vi "test21-RegisterInterruptFromNonCSM.vi"(8 "error in (no error)":errorcluster, 11 "TestCase in":refnum<class "testcase-CSMBroadcast.lvclass">) -> (0 "error out":errorcluster, 3 "TestCase out":refnum<class "testcase-CSMBroadcast.lvclass">)   [LabVIEW 2017, in "testcase-CSMBroadcast.lvclass"]
uses:
  testcase-CSMBroadcast.lvclass
  <vilib>/addons/_JKI Toolkits/VI Tester/TestCase.llb/TestCase.lvclass
  src/user.lib/_NEVSTOP/Communicable State Machine(CSM)/Communicable State Machine.lvlib
  CSM/CSM-Testcase.lvlib
  C:/Program Files (x86)/National Instruments/LabVIEW 2017/vi.lib/addons/_JKI Toolkits/VI Tester/TestCase.llb/TestCase.lvclass
panel:
  out "output cluster":T1
  out "LoopCount":i32
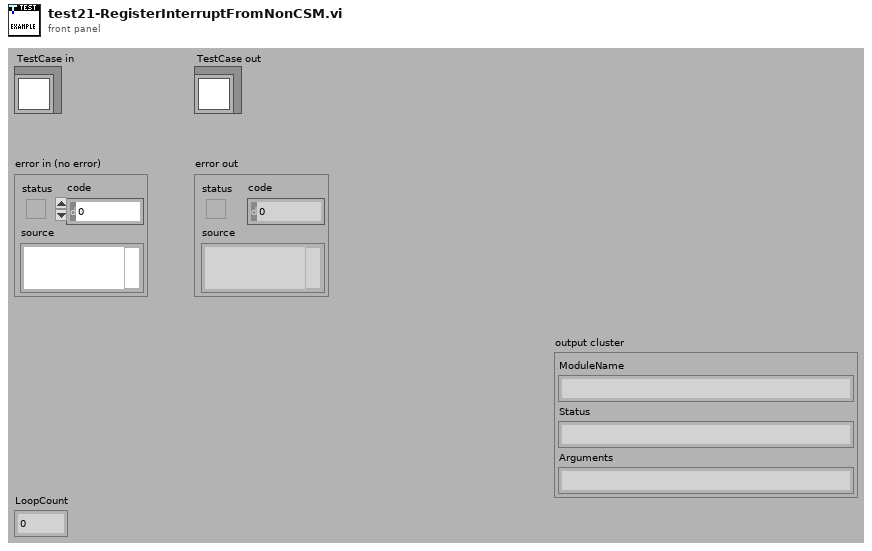
[diagram p1: front panel]
types:
  T1 = cluster{"ModuleName":string, "Status":string, "Arguments":string}
  T2 = cluster{"Status Event":refnum<user-event>, "Interrupt Event":refnum<user-event>}
  T3 = cluster{"cluster":cluster{"ModuleName":string, "Status":string, "Arguments":string}}
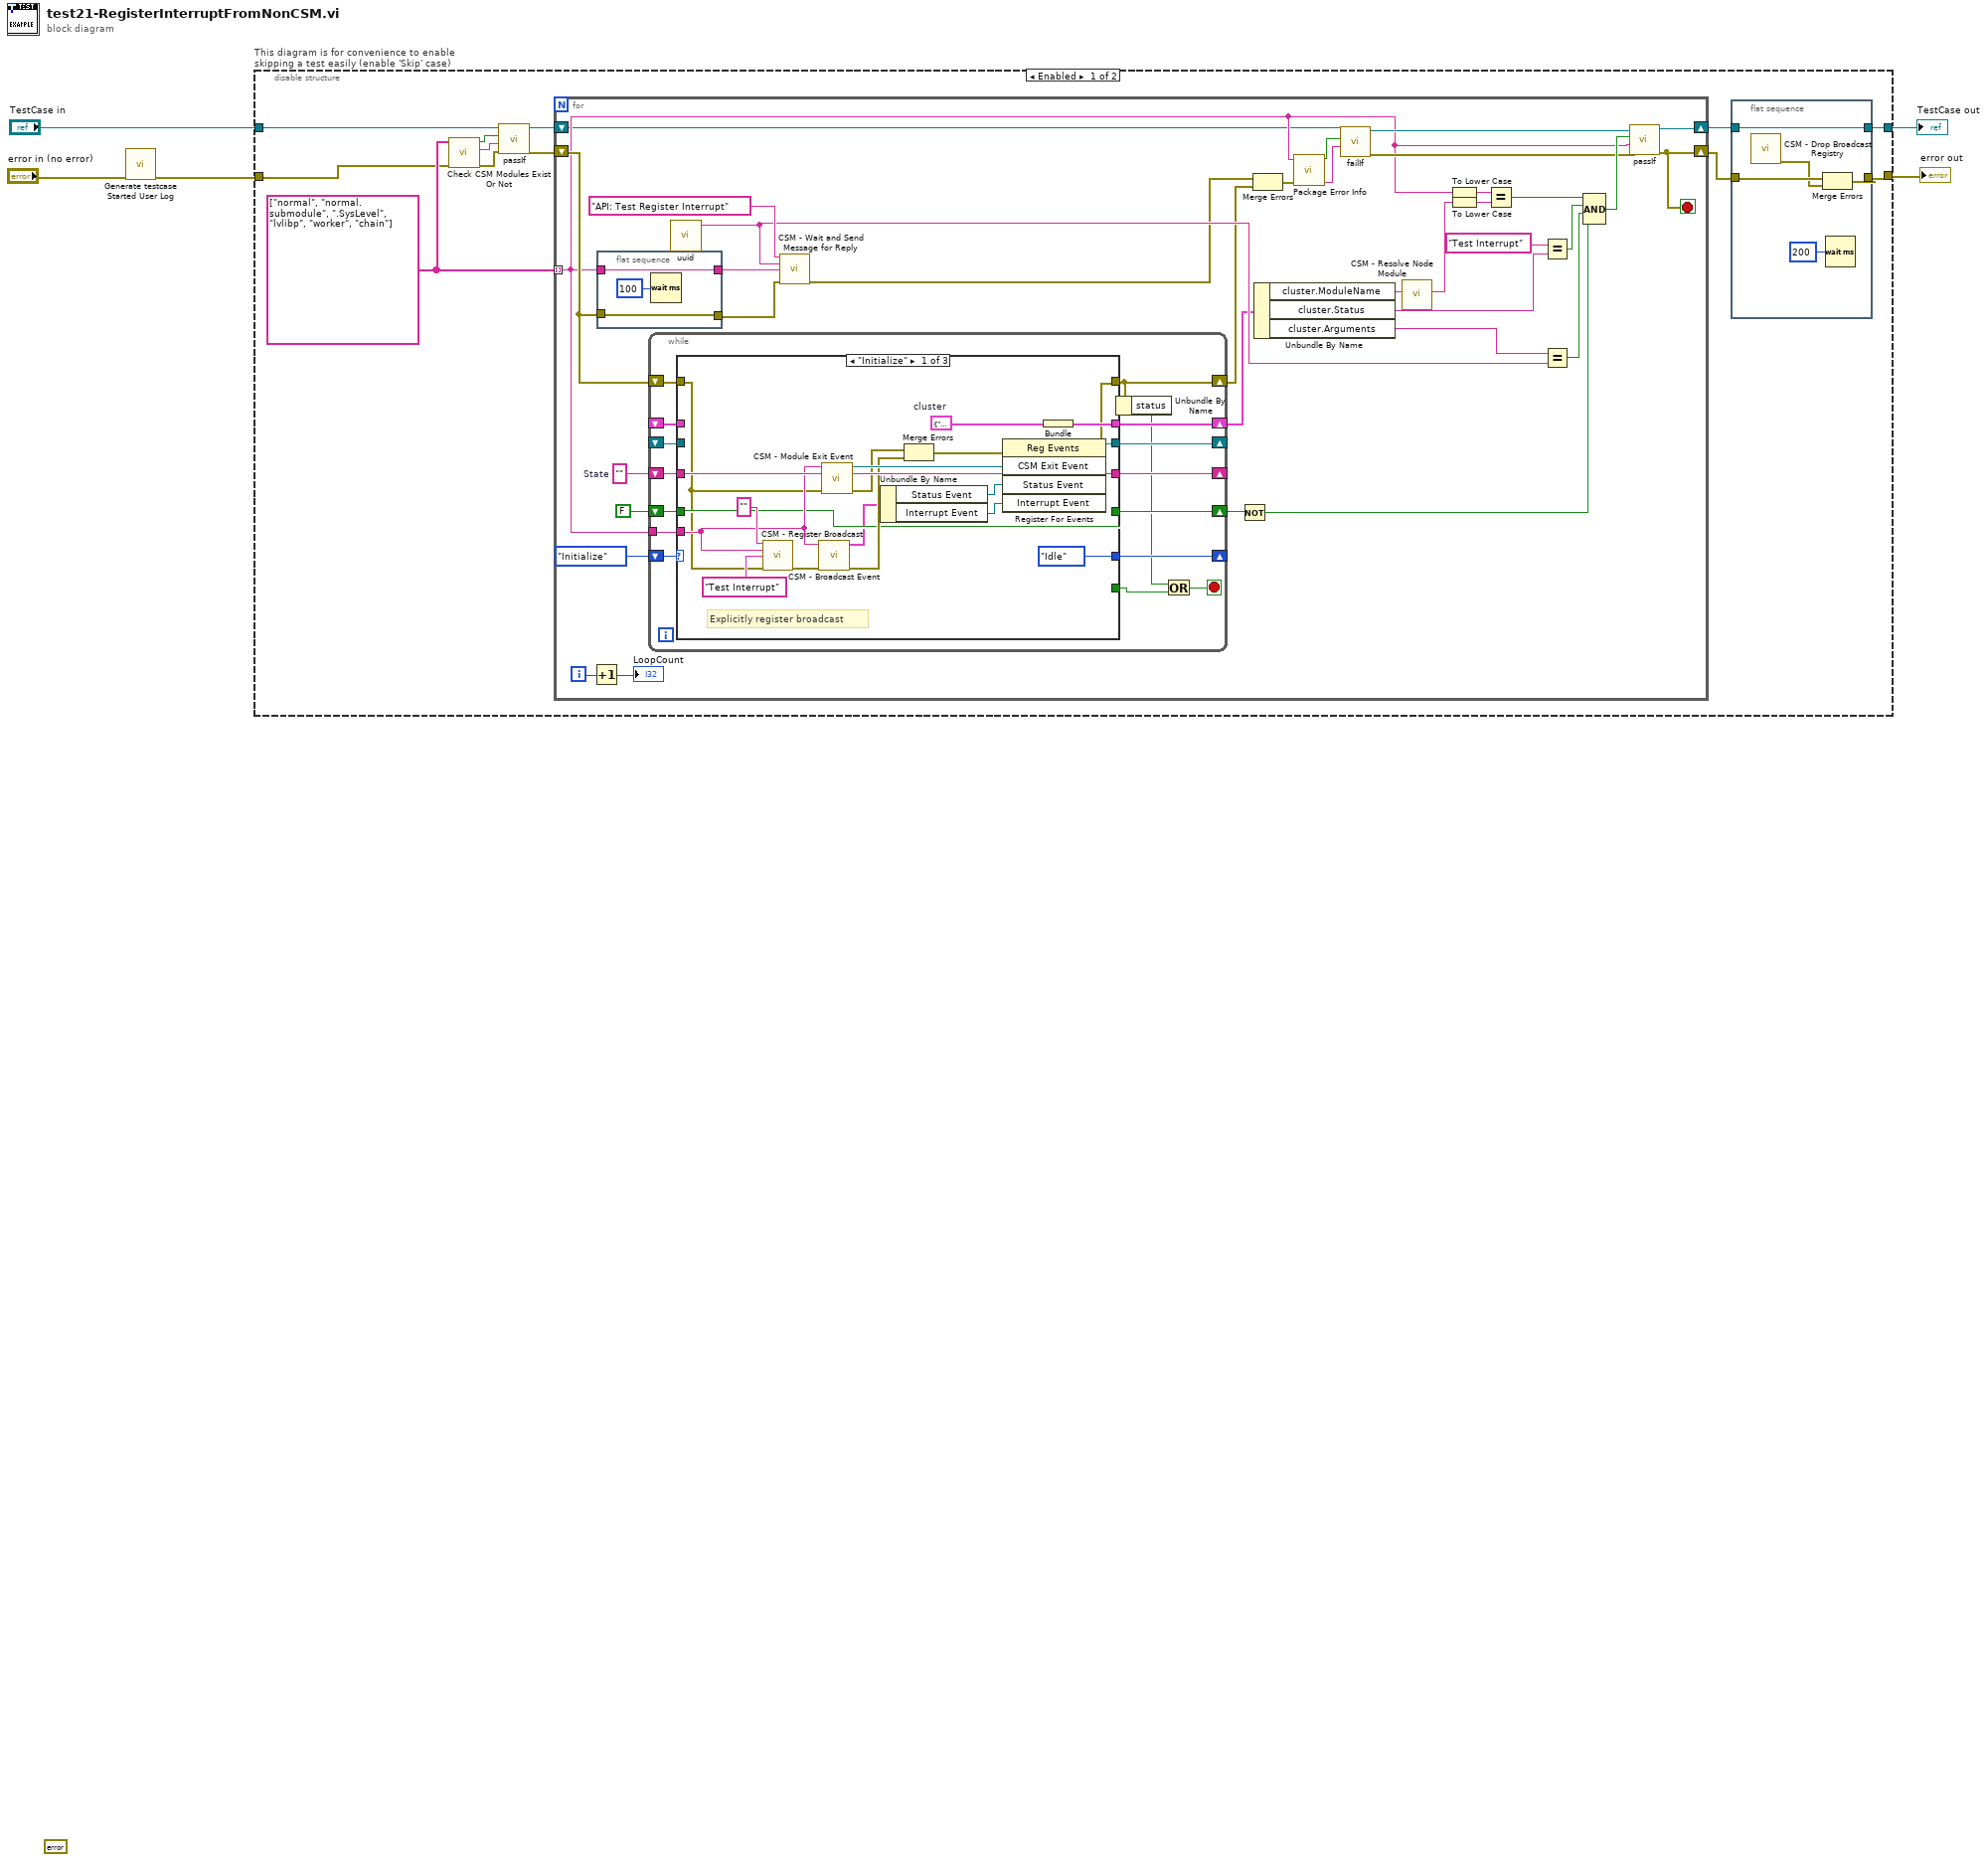
[diagram p0: block diagram]
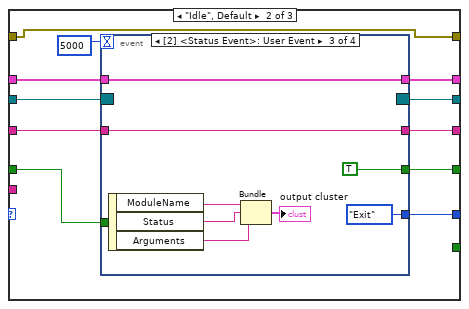
[diagram p2: hidden frame]
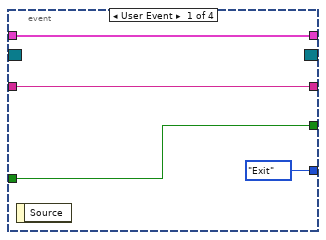
[diagram p3: hidden frame]
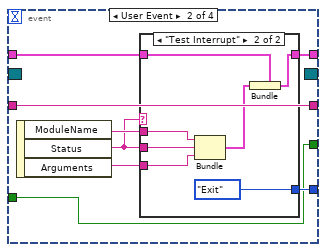
[diagram p4: hidden frame]
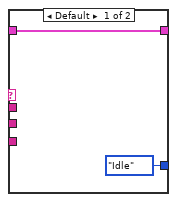
[diagram p5: hidden frame]
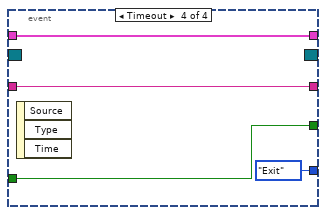
[diagram p6: hidden frame]
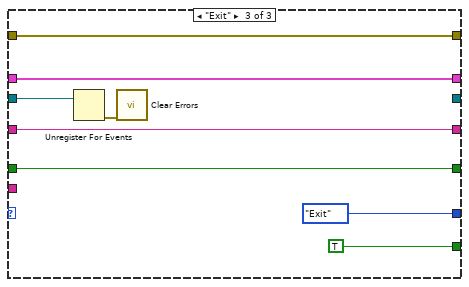
[diagram p7: hidden frame]
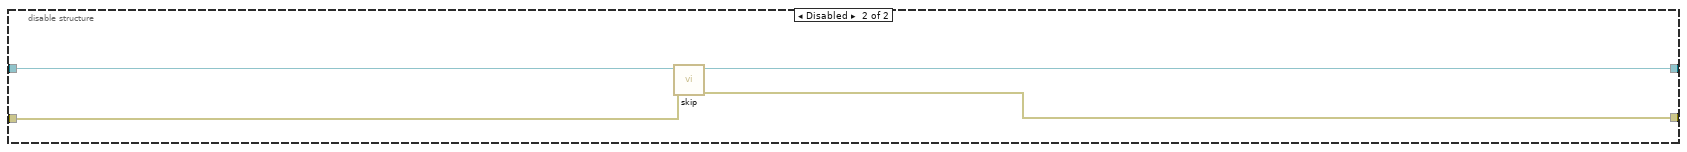
[diagram p8: hidden frame]
diagram:
  (unwired) errorcluster {"status"=FALSE, "code"=0, "source"=""} ("error out")
  n1 = call "Generate testcase Started User Log.vi"("Error In"="error in (no error)") -> ("error out"=w1:errorcluster)  [unwired: 10 in]
  n2 = disable-structure "This diagram is for convenience to enable skipping a test easily (enable 'Skip' case)" shown="Enabled" {
    disable-tunnel: "TestCase in" -> [w12 w151]
    disable-tunnel: [w7 w149] -> w3
    disable-tunnel: [w17 w150] -> w2
    disable-tunnel: w1 -> [w9 w148]
    frame Enabled {
      w13 = string[] ["normal", "normal.submodule", ".SysLevel", "lvlibp", "worker", "chain"]
      n3 = call "Check CSM Modules Exist Or Not.vi"("error in"=w9, "CSM names in"=w13) -> ("error out"=w14:errorcluster, "Debug string"=w15:string, "All Modules Exist?"=w16:bool)  [unwired: 7 in]
      n4 = call-dynamic "passIf.vi"("error in (no error)"=w14, "message (\"\")"=w15, "pass"=w16, "TestCase in"=w12) -> ("error out"=w10:errorcluster, "TestCase out"=w11:refnum<class "testcase-CSMBroadcast.lvclass">)  [unwired: 6 in]
      n5 = for {
        shift-right: [w49] -> w8
        shift-left: w11 -> [w23]
        tunnel: w13 -> [w24] mode=indexing
        shift-right: [w42] -> w6
        shift-left: w10 -> [w32]
        i -> [w44]
        stop <- w42 stop-if-true
        w56 = ""  # State
        n6 = Increment(x=w44) -> (x+1=→"LoopCount":i32)
        n7 = flat-sequence {
          tunnel: w24 -> [w60]
          tunnel: [w60] -> w54
          tunnel: w32 -> [w58]
          tunnel: [w58] -> w33
          frame #0 {
            n8 = Wait (ms)(milliseconds to wait=u32 100) -> ()  [unwired: 1 out]
          }
        }
        n9 = while {
          shift-right: [w75] -> _
          shift-left: enum16{"Idle", "Initialize", "Exit"}."Initialize" -> [w76]
          shift-right: [w73] -> _
          shift-left: w56 -> [w74]
          shift-right: [w72] -> _
          shift-left: _ -> [w71]
          shift-right: [w70] -> w41
          shift-left: _ -> [w69]
          tunnel: w24 -> [w68]
          shift-right: [w67] -> w36
          shift-left: FALSE -> [w66]
          shift-right: [w62] -> w26
          shift-left: w32 -> [w65]
          stop <- w64 stop-if-true
          n10 = case shown="\"Initialize\"" w76 {
            tunnel: [enum16{"Idle", "Initialize", "Exit"}."Idle" w106 enum16{"Idle", "Initialize", "Exit"}."Exit"] -> w75
            tunnel: [_ _ TRUE] -> w63
            tunnel: w74 -> [w94 w104 w145]
            tunnel: [w94 w105 w145] -> w73
            tunnel: [w92 w102 _] -> w72
            tunnel: w71 -> [_ w103 w144]
            tunnel: [w91 w100 w142] -> w70
            tunnel: w69 -> [_ w101 w142]
            tunnel: w68 -> [w84 _ _]
            tunnel: [w81 w98 w141] -> w67
            tunnel: w66 -> [w81 w97 w141]
            tunnel: w65 -> [w79 w96 w140]
            tunnel: [w77 w96 w140] -> w62
            frame "Initialize" {
              w90 = T1 {"ModuleName"="", "Status"="", "Arguments"=""}  # cluster
              # "Explicitly register broadcast"
              n11 = call "CSM - Register Broadcast.vi"("CSM Name(Empty for Broadcast Event)"="", "Source CSM Name (* as Default)"=w84, "Trigger"="Test Interrupt" ("State"), "Error In"=w79) -> ("error out"=w86:errorcluster)  [unwired: 10 in, 1 out]
              n12 = call "CSM - Broadcast Event.vi"("Error In"=w86, "CSM Module"=w84) -> ("error out"=w88:errorcluster, "Broadcast Event"=w80:T2)  [unwired: 7 in, 1 out]
              n13 = call "CSM - Module Exit Event.vi"("Error In"=w79, "Name (\"\" to Use UUID) In"=w84) -> ("error out"=w89:errorcluster, "CSM Exit Event"=w93:refnum<user-event>)  [unwired: 7 in, 1 out]
              n14 = Unbundle By Name(w80) -> ("Status Event"=w83:refnum<user-event>, "Interrupt Event"=w82:refnum<user-event>)
              n15 = Merge Errors(w89, w88) -> (w78:errorcluster)
              n16 = register-events(error in=w78, w93, w83, w82) -> (reference out=w92:refnum<event-registration>, error out=w77:errorcluster)  [unwired: 1 in]
              n17 = Bundle("cluster"=w90) -> (w91:T3)  [unwired: 1 in]
            }
            frame "Idle", Default {
              n18 = event shown="[2] <Status Event>: User Event" {
                selector: w103 -> [_ _ _ _]
                dyn-events: [_ _ _ _] -> w102
                timeout: 5000 -> [_ _ _ _]
                tunnel: [enum16{"Idle", "Initialize", "Exit"}."Exit" w117 enum16{"Idle", "Initialize", "Exit"}."Exit" enum16{"Idle", "Initialize", "Exit"}."Exit"] -> w106
                tunnel: w104 -> [w110 w118 w135 w139]
                tunnel: [w110 w118 w135 w139] -> w105
                tunnel: w101 -> [w108 w114 w134 w138]
                tunnel: [w108 w113 w134 w138] -> w100
                tunnel: [w107 w111 TRUE w136] -> w98
                tunnel: w97 -> [w107 w111 _ w136]
                event User Event {
                  n19 = event-data() -> ()  [unwired: 1 in, 1 out]
                }
                event User Event {
                  n20 = event-data() -> ("ModuleName"=w116:string, "Status"=w112:string, "Arguments"=w115:string)  [unwired: 1 in]
                  n21 = case shown="\"Test Interrupt\"" w112 {
                    tunnel: [enum16{"Idle", "Initialize", "Exit"}."Idle" enum16{"Idle", "Initialize", "Exit"}."Exit"] -> w117
                    tunnel: w116 -> [_ w126]
                    tunnel: w112 -> [_ w125]
                    tunnel: w115 -> [_ w124]
                    tunnel: w114 -> [w120 w123]
                    tunnel: [w120 w121] -> w113
                    frame Default {
                    }
                    frame "Test Interrupt" {
                      n22 = Bundle("ModuleName"=w126, "Status"=w125, "Arguments"=w124) -> (w122:T1)  [unwired: 1 in]
                      n23 = Bundle(cluster=w123, "cluster"=w122) -> (w121:T3)
                    }
                  }
                }
                event User Event {
                  n24 = event-data() -> ("ModuleName"=w131:string, "Status"=w130:string, "Arguments"=w129:string)  [unwired: 1 in]
                  n25 = Bundle("ModuleName"=w131, "Status"=w130, "Arguments"=w129) -> (→"output cluster":T1)  [unwired: 1 in]
                }
                event Timeout {
                  n26 = event-data() -> ()  [unwired: 1 in, 3 out]
                }
              }
            }
            frame "Exit" {
              n27 = Unregister For Events(event registration refnum=w144) -> (error out=w143:errorcluster)  [unwired: 1 in]
              n28 = call <vilib>:"Clear Errors.vi"("error in (no error)"=w143) -> ()  [unwired: 5 in, 2 out]
            }
          }
          n29 = Unbundle By Name(w62) -> ("status"=w61:bool)
          n30 = Or(x=w61, y=w63) -> (x .or. y?=w64:bool)
        }
        n31 = call "uuid.vi"() -> ("UUID"=w51:string)  [unwired: 11 in]
        n32 = call "CSM - Wait and Send Message for Reply.vi"("State"="API: Test Register Interrupt", "Arguments (\"\")"=w51, "Target Module"=w54, "Error In (No Error)"=w33) -> ("error out"=w27:errorcluster)  [unwired: 8 in, 3 out]
        n33 = Not(x=w36) -> (.not. x?=w35:bool)
        n34 = Merge Errors(w27, w26) -> (w25:errorcluster)
        n35 = Unbundle By Name(w41) -> ("cluster.ModuleName"=w39:string, "cluster.Status"=w52:string, "cluster.Arguments"=w50:string)
        n36 = call "Package Error Info.vi"("error in"=w25, "String in"=w24) -> ("packed error info out"=w30:string, "error status"=w31:bool)  [unwired: 8 in]
        n37 = call-dynamic "failIf.vi"("message (\"\")"=w30, "fail"=w31, "TestCase in"=w23) -> ("error out"=w28:errorcluster, "TestCase out"=w29:refnum<class "testcase-CSMBroadcast.lvclass">)  [unwired: 7 in]
        n38 = call "CSM - Resolve Node Module.vi"("Node Name"=w39) -> ("CSM Module Name"=w37:string)  [unwired: 10 in]
        n39 = To Lower Case(string=w24) -> (all lower case string=w40:string)
        n40 = To Lower Case(string=w37) -> (all lower case string=w38:string)
        n41 = Equal?(x=w40, y=w38) -> (x = y?=w48:bool)
        n42 = Equal?(x="Test Interrupt" ("State"), y=w52) -> (x = y?=w47:bool)
        n43 = Equal?(x=w50, y=w51) -> (x = y?=w46:bool)
        n44 = Compound Arithmetic op=AND(w48, w47, w46, w35) -> (w45:bool)
        n45 = call-dynamic "passIf.vi"("error in (no error)"=w28, "message (\"\")"=w24, "pass"=w45, "TestCase in"=w29) -> ("error out"=w42:errorcluster, "TestCase out"=w49:refnum<class "testcase-CSMBroadcast.lvclass">)  [unwired: 6 in]
      }
      n46 = flat-sequence {
        tunnel: w6 -> [w22]
        tunnel: [w21] -> w17
        tunnel: w8 -> [w19]
        tunnel: [w19] -> w7
        frame #0 {
          n47 = call "CSM - Drop Broadcast Registry.vi"() -> ("error out"=w20:errorcluster)  [unwired: 15 in]
          n48 = Merge Errors(w22, w20) -> (w21:errorcluster)
          n49 = Wait (ms)(milliseconds to wait=u32 200) -> ()  [unwired: 1 out]
        }
      }
    }
    frame Disabled {
      # "skip test result while test is under development"
      n50 = call <vilib>:"skip.vi"("error in (no error)"=w148, "TestCase in"=w151) -> ("error out"=w150:errorcluster, "TestCase out"=w149:refnum<class "testcase-CSMBroadcast.lvclass">)  [unwired: 8 in]
    }
  }
  "error out" <- w2
  "TestCase out" <- w3
